vi "GUI_SID4.vi"() -> ()   [LabVIEW 2013]
uses:
  GUI_Template/GUI_master/tcp_new_data_event.ctl
  GUI_Template/GUI_master/tcp new data cluster.ctl
  <vilib>/vision/Image Controls.llb/IMAQ Image.ctl
panel:
  in  "trigger::1":enum16{"Internal", "External"}(ring) caption="trigger"
  in  "pulsewidth::1":dbl caption="Pulse Width (ns)" min=0.0 max=1000000000.0
  in  "gain::1":dbl caption="gain" min=0.0 max=4095.0
  in  "temperature::1":dbl caption="Temperature (C)" min=-40.0 max=20.0
  out "image::1":T1(plugin-control) caption="Intensity"
  in  "acqready::1":enum16{"yes", "no"}(ring)
  in  "stop":bool
  in  "GUIdevice 1":string="PL2-AndorCam"
  out "tcp data event":T2
  out "error IO 2":errorcluster
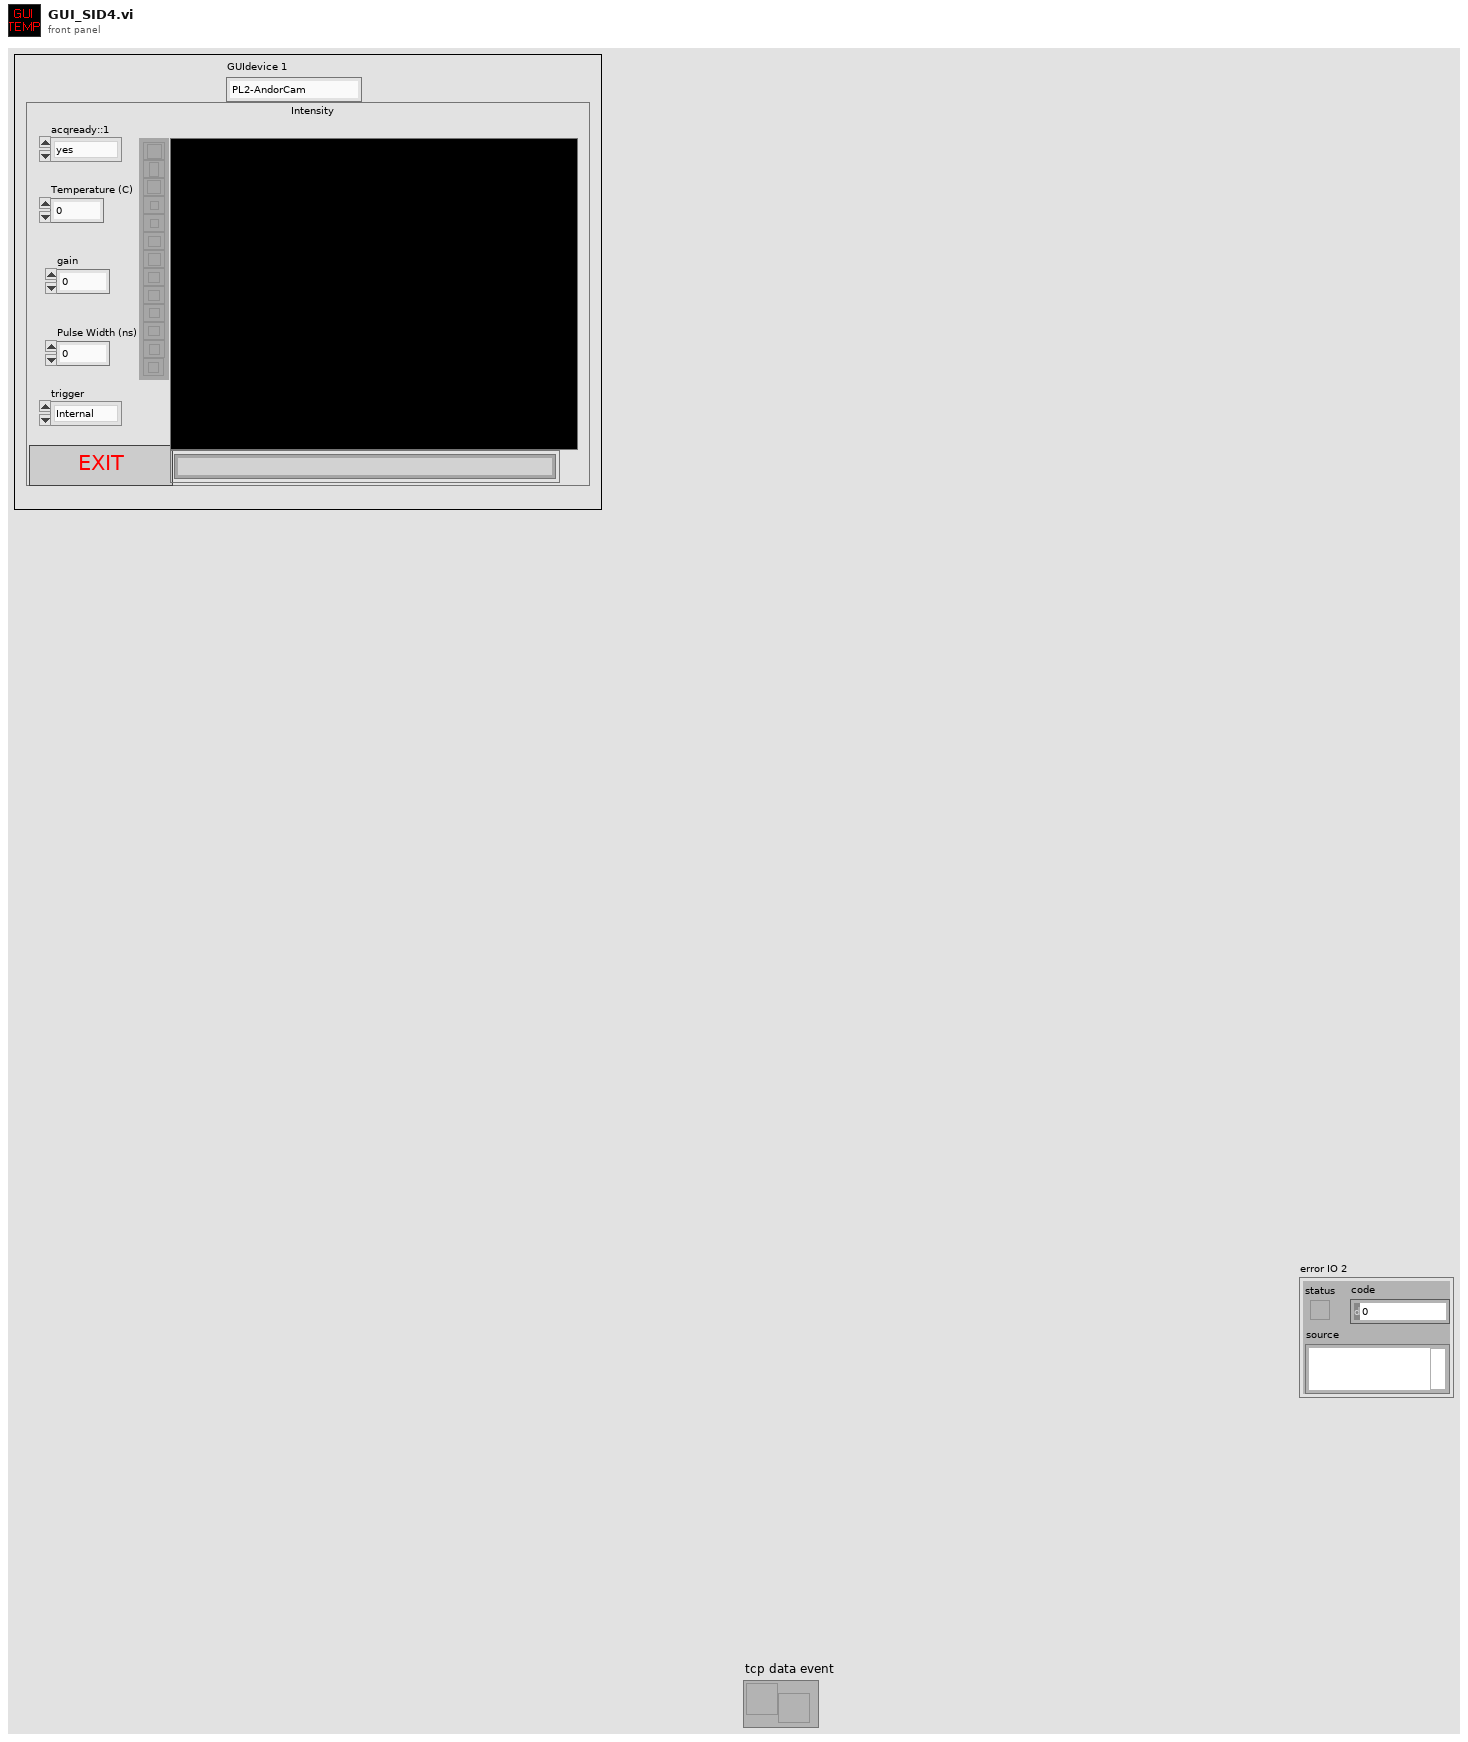
[diagram p1: front panel]
types:
  T1 = typedef "IMAQ Image.ctl" = refnum<image>
  T2 = typedef "tcp_new_data_event.ctl" = refnum<user-event>
  T3 = typedef "tcp new data cluster.ctl" = cluster{"EventEnum":enum16{"new data", "connection status update"}, "Device name":string}
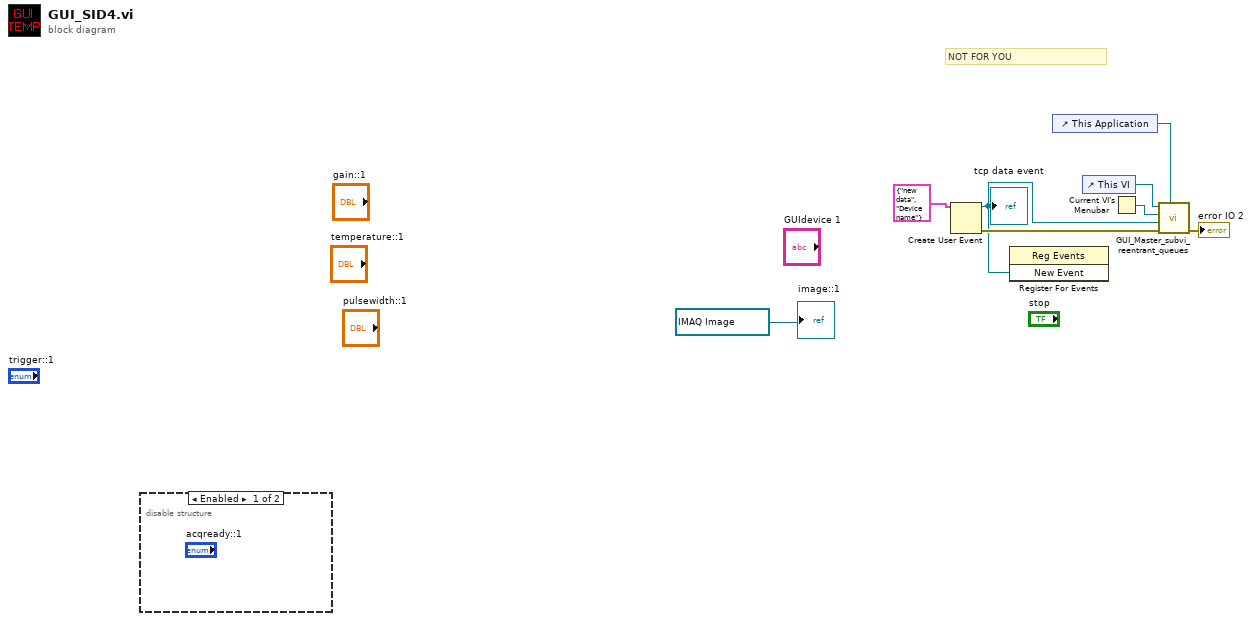
[diagram p0: block diagram]
diagram:
  # "NOT FOR YOU"
  n1 = disable-structure shown="Enabled" {
    frame Enabled {
    }
    frame Disabled {
    }
  }
  n2 = Create User Event(user event datatype=T3 {"EventEnum"=enum."new data", "Device name"="Device name"} ("New Event")) -> (user event=w3:refnum<user-event>, error out=w4:errorcluster)  [unwired: 1 in]
  "tcp data event" <- w3
  n3 = register-events(w3) -> ()  [unwired: 2 in, 2 out]
  n4 = control-ref of="This Application"() -> (w2:refnum<vi>)
  n5 = control-ref of="This VI"() -> (w7:refnum<vi>)
  n6 = Current VI's Menubar() -> (w6:refnum<k9>)
  n7 = call "GUI_Master_subvi_reentrant_queues.vi"("This Application"=w2, "error in (no error)"=w4, "tcp data event"=w3, "Caller menu reference"=w6, "Caller VI ref"=w7) -> ("error out"=→"error IO 2":errorcluster)  [unwired: 6 in]
  "image::1" <- T1 refnum ("image::1")
